vi "Pitch_with_complementary_filter.vi"(1 "ay":i32, 2 "az":i32, 3 "% Gyro":dbl=1.0 format="%#_13g", 4 "*pitch":dbl) -> (0 "pitch":i32)   [LabVIEW 2015]
doc: "pitch = atan2(ax,sqrt((ay*ay)+(az*az)))*(180/pi)"
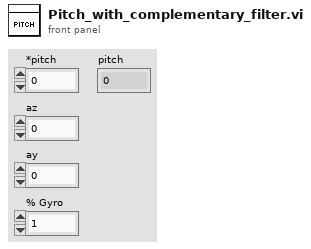
[diagram p1: front panel]
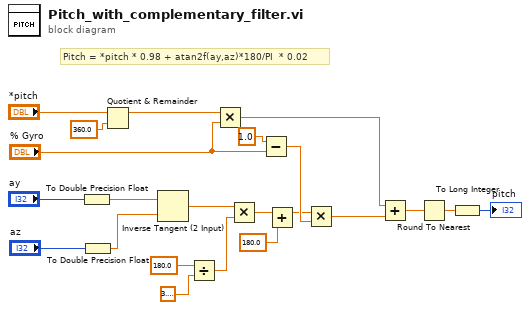
[diagram p0: block diagram]
diagram:
  # "Pitch = *pitch * 0.98 + atan2f(ay,az)*180/PI  * 0.02"
  n1 = To Double Precision Float(number="ay") -> (double precision float=w13:dbl)
  n2 = To Double Precision Float(number="az") -> (double precision float=w12:dbl)
  n3 = Quotient & Remainder(x="*pitch", y=360.0) -> (x-y*floor(x/y)=w3:dbl)  [unwired: 1 out]
  n4 = Inverse Tangent (2 Input)(1:w12, 2:w13) -> (0:w22:dbl)
  n5 = Divide(x=180.0, y=3.141592653589793) -> (x/y=w19:dbl)
  n6 = Multiply(x=w3, y="% Gyro") -> (x*y=w15:dbl)
  n7 = Multiply(x=w22, y=w19) -> (x*y=w16:dbl)
  n8 = Subtract(x=1.0, y="% Gyro") -> (x-y=w7:dbl)
  n9 = Add(x=w16, y=180.0) -> (x+y=w2:dbl)
  n10 = Multiply(x=w2, y=w7) -> (x*y=w14:dbl)
  n11 = Add(x=w15, y=w14) -> (x+y=w6:dbl)
  n12 = Round To Nearest(number=w6) -> (nearest integer value=w11:dbl)
  n13 = To Long Integer(number=w11) -> (32bit integer=→"pitch":i32)
